vi "LD2018_ブロック崩し_反射処理.vi"(0 "接触点":i32, 1 "PADDLE座標":T2, 2 "Ball座標":T1, 5 "角度入力":dbl, 7 "方向入力":i32, 9 "Combo中入力":bool, 11 "Play中入力":bool, 12 "残機入力":i32) -> (6 "角度出力":dbl, 8 "方向出力":i32, 10 "Combo中出力":bool, 14 "残機出力":i32, 15 "Play中出力":bool)   [LabVIEW 2016]
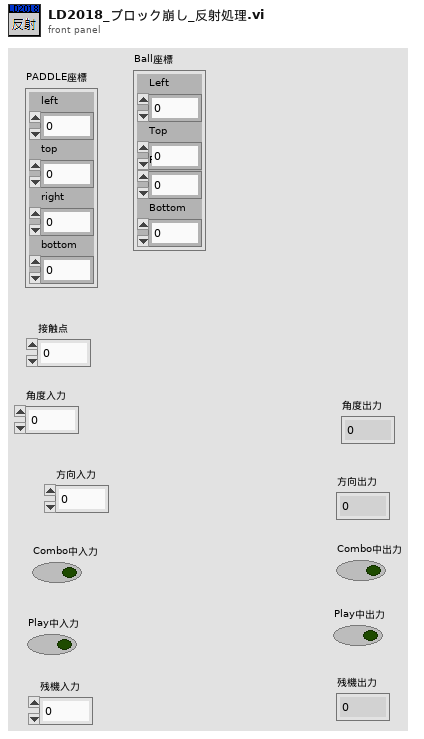
[diagram p1: front panel]
types:
  T1 = cluster{"Left":dbl, "Top":dbl, "Right":dbl, "Bottom":dbl}
  T2 = cluster{"left":i16, "top":i16, "right":i16, "bottom":i16}
  T3 = cluster{"Left":i16, "Top":i16, "Right":i16, "Bottom":i16}
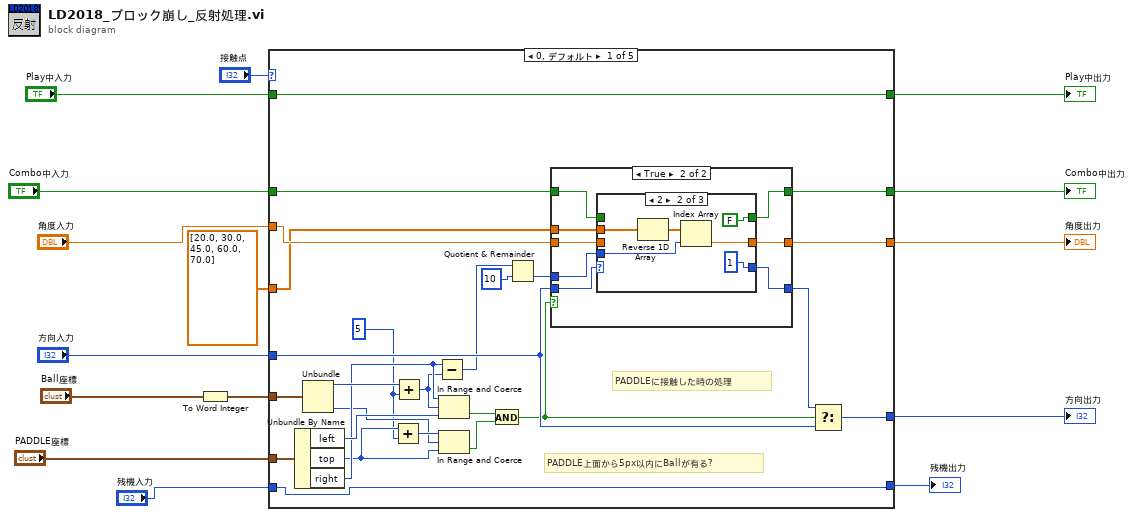
[diagram p0: block diagram]
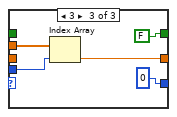
[diagram p4: hidden frame]
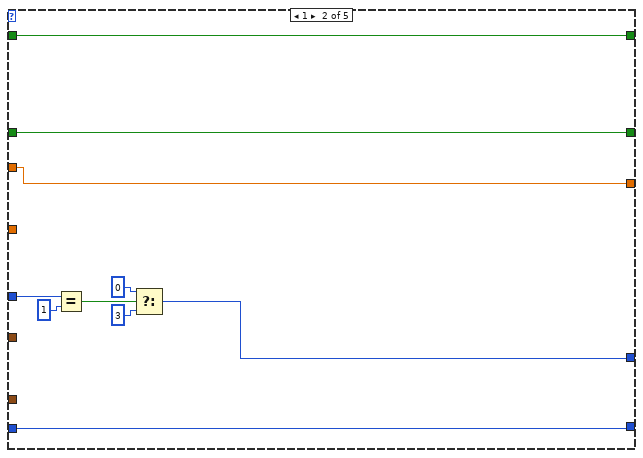
[diagram p5: hidden frame]
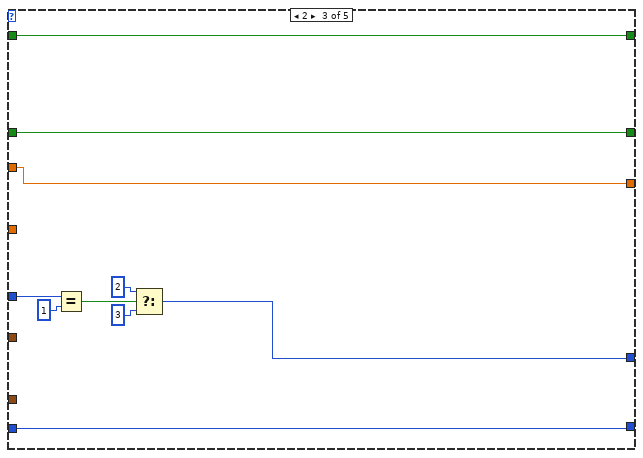
[diagram p6: hidden frame]
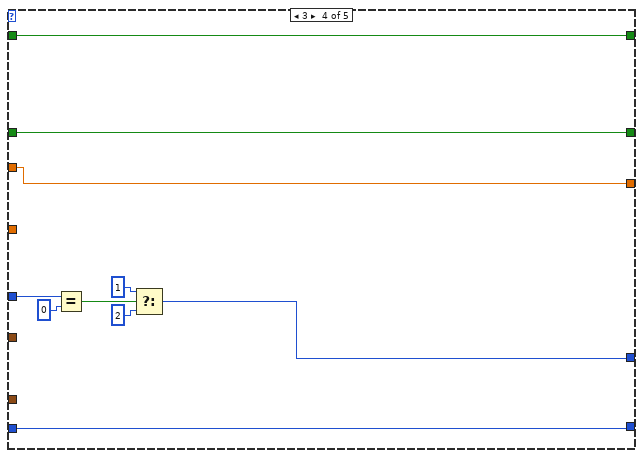
[diagram p7: hidden frame]
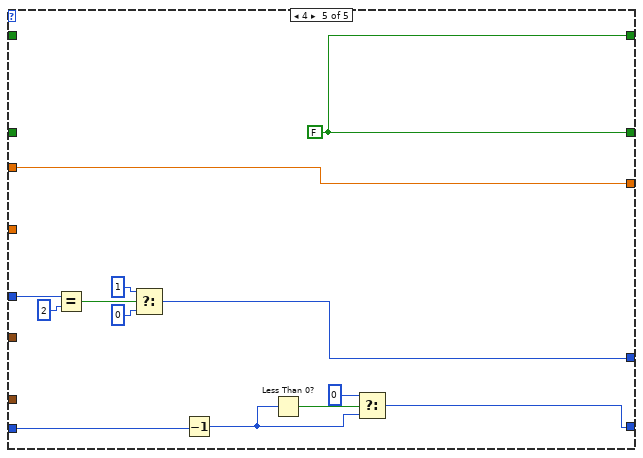
[diagram p8: hidden frame]
diagram:
  n1 = To Word Integer(number="Ball座標") -> (16bit integer=w3:T3)
  n2 = case shown="0, デフォルト" "接触点" {
    tunnel: [w35 w74 w86 w91 w104] -> w8
    tunnel: "方向入力" -> [w34 w73 w83 w96 w109]
    tunnel: "PADDLE座標" -> [w41 _ _ _ _]
    tunnel: w3 -> [w40 _ _ _ _]
    tunnel: "角度入力" -> [w31 w70 w80 w90 w103]
    tunnel: [w25 w70 w80 w90 w103] -> w7
    tunnel: dbl[] [20.0, 30.0, 45.0, 60.0, 70.0] -> [w26 _ _ _ _]
    tunnel: "Combo中入力" -> [w24 w69 w79 w89 _]
    tunnel: [w23 w69 w79 w89 w102] -> w10
    tunnel: "Play中入力" -> [w22 w68 w78 w88 _]
    tunnel: [w22 w68 w78 w88 w102] -> w15
    tunnel: "残機入力" -> [w16 w67 w77 w87 w101]
    tunnel: [w16 w67 w77 w87 w97] -> w1
    frame 0, Default {
      w17 = i16 5 ("y")
      # "PADDLE上面から5px以内にBallが有る?"
      # "PADDLEに接触した時の処理"
      n3 = Unbundle By Name(w41) -> ("left"=w38:i16, "top"=w20:i16, "right"=w33:i16)
      n4 = Unbundle(w40) -> ("Left"=w39:i16, "Bottom"=w19:i16)  [unwired: 2 out]
      n5 = Add(x=w20, y=w17) -> (x+y=w21:i16)
      n6 = Add(x=w39, y=w17) -> (x+y=w32:i16)
      n7 = Subtract(x=w33, y=w32) -> (x-y=w29:i16)
      n8 = In Range and Coerce(upper limit=w33, x=w32, lower limit=w38) -> (In Range?=w37:bool)  [unwired: 1 out]
      n9 = In Range and Coerce(upper limit=w21, x=w19, lower limit=w20) -> (In Range?=w18:bool)  [unwired: 1 out]
      n10 = And(x=w37, y=w18) -> (x .and. y?=w30:bool)
      n11 = Quotient & Remainder(x=w29, y=i16 10) -> (floor(x/y)=w27:i16)  [unwired: 1 out]
      n12 = case shown="TRUE" w30 {
        tunnel: [w43 w52] -> w36
        tunnel: w34 -> [w43 w51]
        tunnel: w31 -> [w44 w50]
        tunnel: [w44 w49] -> w25
        tunnel: w26 -> [_ w48]
        tunnel: w27 -> [_ w47]
        tunnel: w24 -> [w42 w46]
        tunnel: [w42 w45] -> w23
        frame False {
        }
        frame True {
          n13 = case shown="2" w51 {
            selector: w51 -> [w55 _ _]
            tunnel: [w55 i16 1 ("y") i16 0] -> w52
            tunnel: w50 -> [w54 _ _]
            tunnel: [w54 w59 w64] -> w49
            tunnel: w48 -> [_ w58 w63]
            tunnel: w47 -> [_ w60 w65]
            tunnel: w46 -> [w53 _ _]
            tunnel: [w53 FALSE FALSE] -> w45
            frame 0, Default {
            }
            frame 2 {
              n14 = Reverse 1D Array(array=w58) -> (reversed array=w57:dbl[])
              n15 = Index Array(array=w57, index=w60) -> (element=w59:dbl)
            }
            frame 3 {
              n16 = Index Array(array=w63, index=w65) -> (element=w64:dbl)
            }
          }
        }
      }
      n17 = Select(t=w36, s=w30, f=w34) -> (s? t:f=w35:i32)
    }
    frame 1 {
      n18 = Equal?(x=w73, y=1) -> (x = y?=w71:bool)
      n19 = Select(t=0, s=w71, f=3) -> (s? t:f=w74:i32)
    }
    frame 2 {
      n20 = Equal?(x=w83, y=1 ("f")) -> (x = y?=w81:bool)
      n21 = Select(t=2, s=w81, f=3) -> (s? t:f=w86:i32)
    }
    frame 3 {
      n22 = Equal?(x=w96, y=0) -> (x = y?=w94:bool)
      n23 = Select(t=1 ("y"), s=w94, f=2 ("y")) -> (s? t:f=w91:i32)
    }
    frame 4 {
      w102 = FALSE
      n24 = Equal?(x=w109, y=2) -> (x = y?=w107:bool)
      n25 = Select(t=1 ("y"), s=w107, f=0 ("y")) -> (s? t:f=w104:i32)
      n26 = Decrement(x=w101) -> (x-1=w99:i32)
      n27 = Less Than 0?(x=w99) -> (x < 0?=w100:bool)
      n28 = Select(t=0, s=w100, f=w99) -> (s? t:f=w97:i32)
    }
  }
  "Play中出力" <- w15
  "Combo中出力" <- w10
  "方向出力" <- w8
  "角度出力" <- w7
  "残機出力" <- w1
